vi "Wave-Check Riff.vi"(8 "error in (no error)":errorcluster, 10 "ID":string="WAVE", 11 "refnum":refnum<file>) -> (0 "error out":errorcluster, 2 "is OK?":bool, 3 "refnum out":refnum<file>)   [LabVIEW 2020]
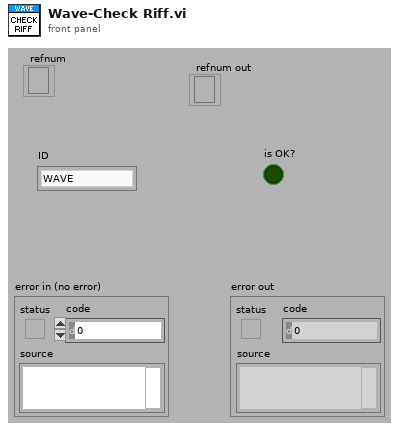
[diagram p1: front panel]
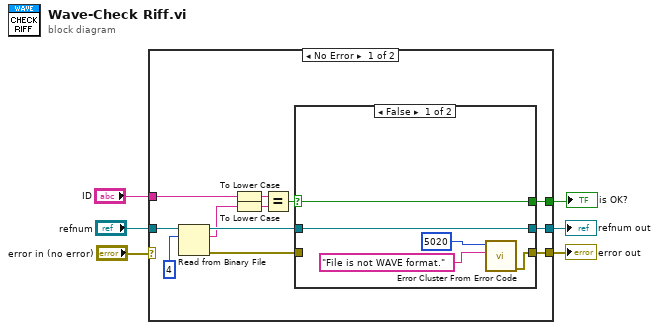
[diagram p0: block diagram]
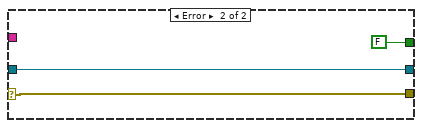
[diagram p3: hidden frame]
diagram:
  n1 = case shown="No Error" "error in (no error)" {
    selector: "error in (no error)" -> [_ w27]
    tunnel: "refnum" -> [w18 w29]
    tunnel: [w14 w29] -> w5
    tunnel: [w13 w27] -> w4
    tunnel: "ID" -> [w12 _]
    tunnel: [w9 FALSE] -> w2
    frame No Error {
      n2 = Read from Binary File(10:4, 11:w18) -> (0:w16:errorcluster, 2:w11:string, 3:w15:refnum<file>)  [unwired: 4 in, 1 out]
      n3 = To Lower Case(string=w12) -> (all lower case string=w8:string)
      n4 = To Lower Case(string=w11) -> (all lower case string=w7:string)
      n5 = Equal?(x=w8, y=w7) -> (x = y?=w10:bool)
      n6 = case shown="False" w10 {
        selector: w10 -> [w22 w26]
        tunnel: w16 -> [_ w24]
        tunnel: w15 -> [w23 w25]
        tunnel: [w23 w25] -> w14
        tunnel: [w21 w24] -> w13
        tunnel: [w22 w26] -> w9
        frame False {
          n7 = call <vilib>:"Error Cluster From Error Code.vi"("error message (\"\")"="File is not WAVE format." ("source"), "error code (0)"=5020) -> ("error out"=w21:errorcluster)  [unwired: 7 in]
        }
        frame True {
        }
      }
    }
    frame Error {
    }
  }
  "error out" <- w4
  "refnum out" <- w5
  "is OK?" <- w2
